vi "MakeTimestampedSegmentExample.vi"() -> ()   [LabVIEW 2015]
uses:
  <vilib>/MDSplus/Library/MDSplus.lvlib
panel:
  out "output array":dbl[][](array[numeric])
  out "MDSplus error":errorcluster
  in  "Samples per segment":i32=100
  in  "Sampling time [ms]":i32=10
  in  "stop":bool
  in  "Phase":dbl
  in  "Amplitude":dbl=5.0
  in  "Frequency":dbl=0.01
  in  "Node path":string
  in  "Run number":i32
  in  "Tree name":string
  # "Before running this example make sure to set the Tree name, Run number and Node path to meaningful values.\nNote that the example does not create a tree structure for you. If a signal (?) node is not already present when you call it, the example will fail."
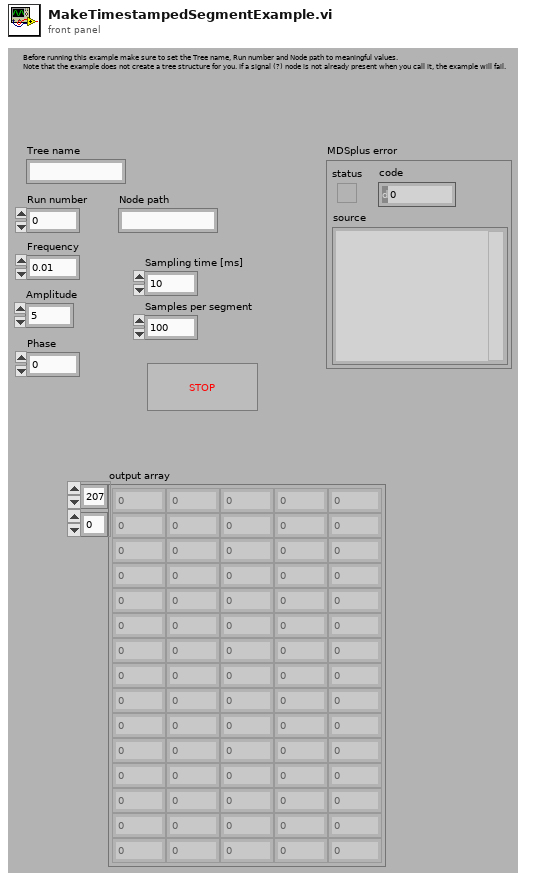
[diagram p1: front panel]
types:
  T1 = cluster{"Data channels":dbl[][], "Timestamps":timestamp[]}
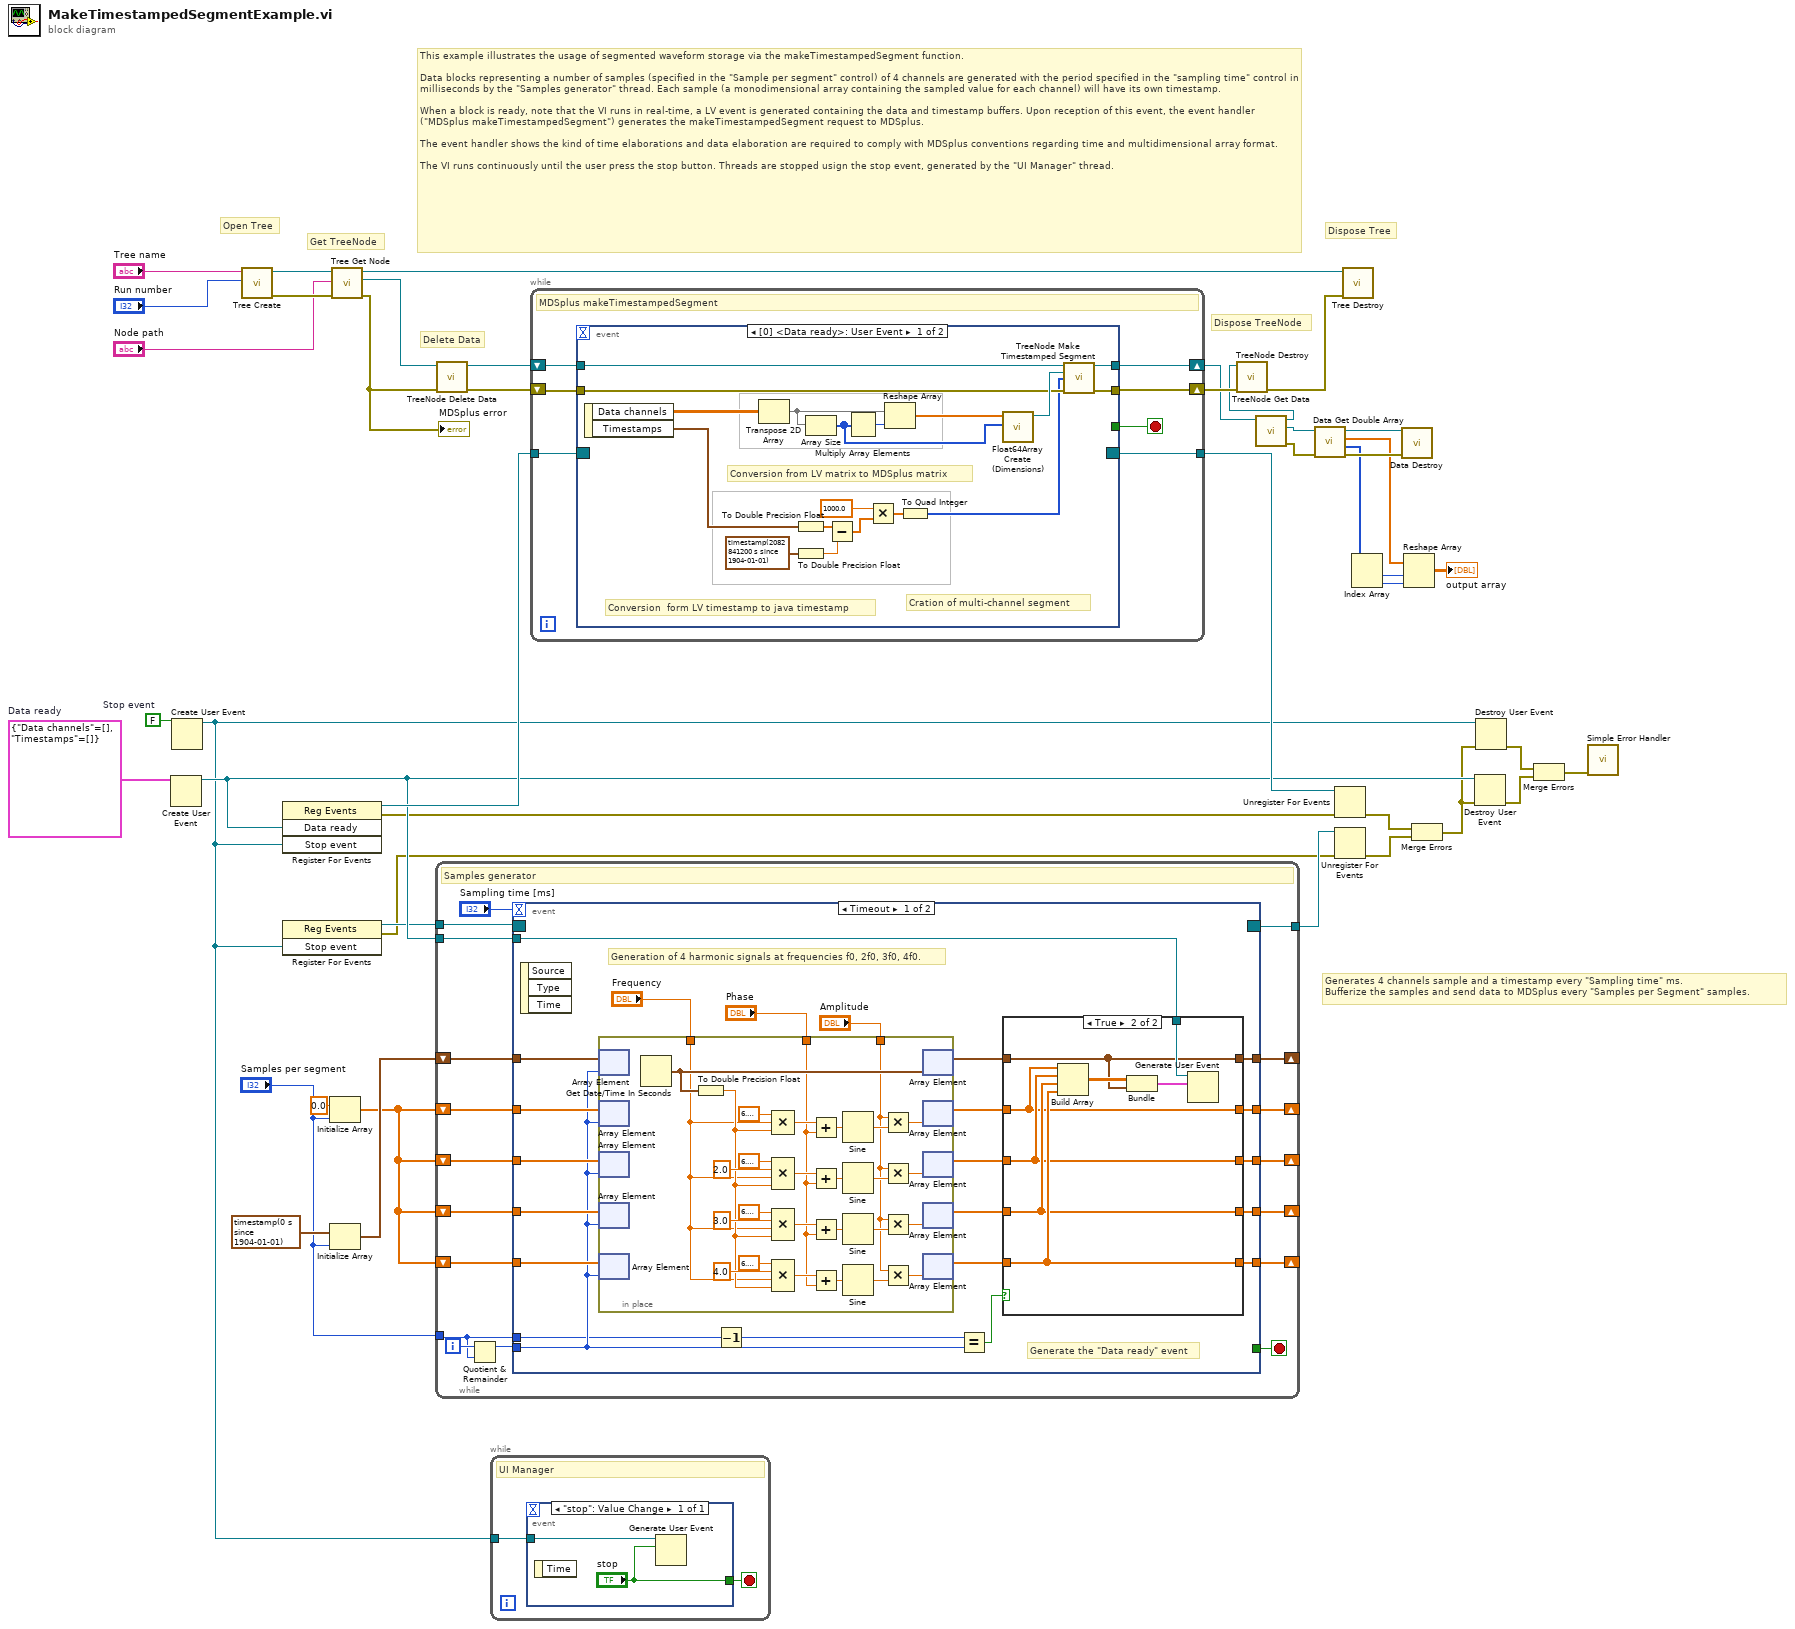
[diagram p0: block diagram]
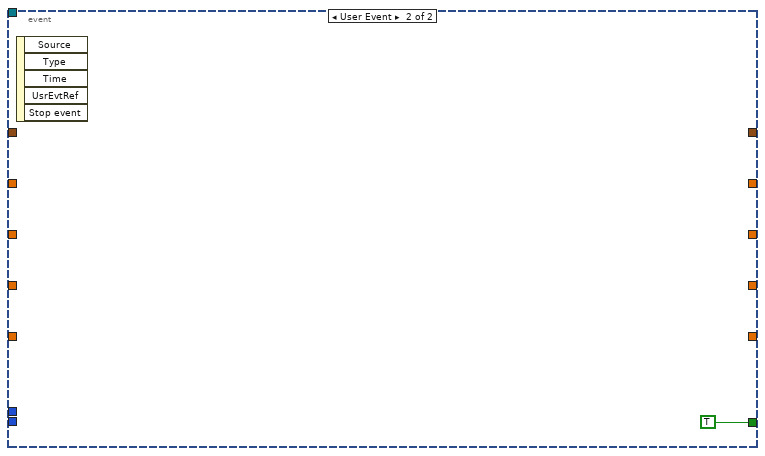
[diagram p3: hidden frame]
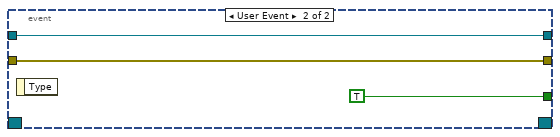
[diagram p4: hidden frame]
diagram:
  w29 = T1 {"Data channels"=[], "Timestamps"=[]}  # Data ready
  w32 = FALSE  # Stop event
  # "Generates 4 channels sample and a timestamp every \"Sampling time\" ms.\nBufferize the samples and send data to MDSplus every \"Samples per Segment\" samples."
  # "Dispose TreeNode"
  # "Delete Data"
  # "Get TreeNode"
  # "This example illustrates the usage of segmented waveform storage via the makeTimestampedSegment function.\n\nData blocks representing a number of samples (specified in the \"Sample per segment\" control) of 4 channels are generated with the period specified in the \"sampling time\" control in milliseconds by the \"Samples generator\" thread. Each sample (a monodimensional array containing the sampled value for each channel) will have its own timestamp.\n\nWhen a block is ready, note that the VI runs in real-time, a LV event is generated containing the data and timestamp buffers. Upon reception of this event, the event handler (\"MDSplus makeTimestampedSegment\") generates the makeTimestampedSegment request to MDSplus.\n\nThe event handler shows the kind of time elaborations and data elaboration are required to comply with MDSplus conventions regarding time and multidimensional array format.\n\nThe VI runs continuously until the user press the stop button. Threads are stopped usign the stop event, generated by the \"UI Manager\" thread."
  # "Dispose Tree"
  # "Open Tree"
  n1 = Create User Event(user event datatype=w29) -> (user event=w33:refnum<user-event>)  [unwired: 1 in, 1 out]
  n2 = Create User Event(user event datatype=w32) -> (user event=w21:refnum<user-event>)  [unwired: 1 in, 1 out]
  n3 = call <vilib>:"Tree Create.vi"("Shot"="Run number", "Name"="Tree name") -> ("error out"=w40:errorcluster, "Tree DVR out"=w42:refnum<data-value>)  [unwired: 8 in]
  n4 = register-events(w33, w21) -> (reference out=w35:refnum<event-registration>, error out=w28:errorcluster)  [unwired: 2 in]
  n5 = register-events(w21) -> (reference out=w25:refnum<event-registration>, error out=w23:errorcluster)  [unwired: 2 in]
  n6 = Initialize Array(0.0 ("phase"), "Samples per segment") -> (w19:dbl[])
  n7 = Initialize Array(timestamp(0 s since 1904-01-01), "Samples per segment") -> (w20:timestamp[])
  n8 = call <vilib>:"Tree Get Node.vi"("error in (no error)"=w40, "Path"="Node path", "Tree DVR in"=w42) -> ("error out"=w13:errorcluster, "Node out"=w37:refnum<data-value>, "Tree DVR out"=w41:refnum<data-value>)  [unwired: 6 in]
  "MDSplus error" <- w13
  n9 = while {
    tunnel: w33 -> [w62]
    shift-right: [w49] -> _
    shift-left: w20 -> [w61]
    shift-right: [w48] -> _
    shift-left: w19 -> [w60]
    shift-right: [w51] -> _
    shift-left: w19 -> [w58]
    shift-right: [w50] -> _
    shift-left: w19 -> [w59]
    shift-right: [w52] -> _
    shift-left: w19 -> [w57]
    tunnel: "Samples per segment" -> [w53]
    tunnel: w25 -> [w47]
    tunnel: [w45] -> w24
    i -> [w56]
    stop <- w46 stop-if-true
    # "Samples generator"
    n10 = Quotient & Remainder(x=w56, y=w53) -> (x-y*floor(x/y)=w55:i32)  [unwired: 1 out]
    n11 = event shown="[0] Timeout" {
      selector: w47 -> [_ _]
      dyn-events: [_ _] -> w45
      timeout: "Sampling time [ms]" -> [_ _]
      tunnel: w62 -> [w80 _]
      tunnel: w61 -> [w79 _]
      tunnel: w60 -> [w78 _]
      tunnel: w59 -> [w77 _]
      tunnel: w58 -> [w76 _]
      tunnel: w57 -> [w75 _]
      tunnel: w55 -> [w71 _]
      tunnel: w53 -> [w64 _]
      tunnel: [w69 _] -> w52
      tunnel: [w68 _] -> w51
      tunnel: [w67 _] -> w50
      tunnel: [w66 _] -> w49
      tunnel: [w65 _] -> w48
      tunnel: [_ TRUE] -> w46
      event Timeout {
        # "Generate the \"Data ready\" event"
        # "Generation of 4 harmonic signals at frequencies f0, 2f0, 3f0, 4f0."
        n12 = event-data() -> ()  [unwired: 1 in, 3 out]
        n13 = in-place {
          in-place-border: "Frequency" -> [w99]
          in-place-border: "Amplitude" -> [w101]
          in-place-border: "Phase" -> [w100]
          n14 = in-place-array #1(w79, w71) -> ()  [unwired: 1 out]
          n15 = in-place-array #2(w78, w71) -> ()  [unwired: 1 out]
          n16 = in-place-array #3(w77, w71) -> ()  [unwired: 1 out]
          n17 = in-place-array #4(w76, w71) -> ()  [unwired: 1 out]
          n18 = in-place-array #5(w75, w71) -> ()  [unwired: 1 out]
          n19 = Get Date/Time In Seconds() -> (seconds since 1Jan1904=w122:timestamp)
          n20 = To Double Precision Float(number=w122) -> (double precision float=w105:dbl)
          n21 = Compound Arithmetic op=MULTIPLY(6.283185307179586, w99, w105) -> (w125:dbl)
          n22 = Compound Arithmetic op=MULTIPLY(6.283185307179586, 2.0 ("value"), w99, w105) -> (w119:dbl)
          n23 = Compound Arithmetic op=MULTIPLY(6.283185307179586, 3.0 ("value"), w99, w105) -> (w114:dbl)
          n24 = Compound Arithmetic op=MULTIPLY(6.283185307179586, 4.0 ("value"), w99, w105) -> (w109:dbl)
          n25 = Add(x=w125, y=w100) -> (x+y=w126:dbl)
          n26 = Add(x=w119, y=w100) -> (x+y=w120:dbl)
          n27 = Add(x=w114, y=w100) -> (x+y=w115:dbl)
          n28 = Add(x=w109, y=w100) -> (x+y=w110:dbl)
          n29 = Sine(x=w126) -> (sin(x)=w124:dbl)
          n30 = Sine(x=w120) -> (sin(x)=w118:dbl)
          n31 = Sine(x=w115) -> (sin(x)=w113:dbl)
          n32 = Sine(x=w110) -> (sin(x)=w108:dbl)
          n33 = Multiply(x=w101, y=w124) -> (x*y=w121:dbl)
          n34 = Multiply(x=w101, y=w118) -> (x*y=w104:dbl)
          n35 = Multiply(x=w101, y=w113) -> (x*y=w103:dbl)
          n36 = Multiply(x=w101, y=w108) -> (x*y=w102:dbl)
          n37 = in-place-array #1(w122) -> (w81:timestamp[])  [unwired: 1 out]
          n38 = in-place-array #2(w121) -> (w82:dbl[])  [unwired: 1 out]
          n39 = in-place-array #3(w104) -> (w83:dbl[])  [unwired: 1 out]
          n40 = in-place-array #4(w103) -> (w84:dbl[])  [unwired: 1 out]
          n41 = in-place-array #5(w102) -> (w85:dbl[])  [unwired: 1 out]
        }
        n42 = Decrement(x=w64) -> (x-1=w63:i32)
        n43 = Equal?(x=w63, y=w71) -> (x = y?=w70:bool)
        n44 = case shown="True" w70 {
          tunnel: w85 -> [w86 w95]
          tunnel: w84 -> [w87 w94]
          tunnel: w83 -> [w88 w93]
          tunnel: w82 -> [w89 w91]
          tunnel: w81 -> [w90 w92]
          tunnel: w80 -> [_ w96]
          tunnel: [w86 w95] -> w69
          tunnel: [w87 w94] -> w68
          tunnel: [w88 w93] -> w67
          tunnel: [w90 w92] -> w66
          tunnel: [w89 w91] -> w65
          frame False {
          }
          frame True {
            n45 = Build Array(w91, w93, w94, w95) -> (w98:dbl[][])
            n46 = Bundle(w98, w92) -> (w97:cluster{dbl[][], timestamp[]})  [unwired: 1 in]
            n47 = Generate User Event(user event=w96, event data cluster=w97) -> ()  [unwired: 2 in, 2 out]
          }
        }
      }
      event User Event {
        n48 = event-data() -> ()  [unwired: 1 in, 5 out]
      }
    }
  }
  n49 = call <vilib>:"TreeNode Delete Data.vi"("error in (no error)"=w13, "TreeNode DVR in"=w37) -> ("error out"=w31:errorcluster, "TreeNode DVR out"=w36:refnum<data-value>)  [unwired: 8 in]
  n50 = while {
    tunnel: w21 -> [w128]
    stop <- w129 stop-if-true
    # "UI Manager"
    n51 = event shown="[0] \"stop\": Value Change" {
      selector: _ -> [_]
      dyn-events: _ -> [_]
      timeout: _ -> [_]
      tunnel: ["stop"] -> w129
      tunnel: w128 -> [w130]
      event "stop": Value Change {
        n52 = event-data() -> ()  [unwired: 1 in, 1 out]
        n53 = Generate User Event(user event=w130, event data cluster="stop") -> ()  [unwired: 2 in, 2 out]
      }
    }
  }
  n54 = while {
    shift-right: [w135] -> w11
    shift-left: w36 -> [w136]
    shift-right: [w132] -> w30
    shift-left: w31 -> [w133]
    tunnel: w35 -> [w138]
    tunnel: [w137] -> w34
    stop <- w134 stop-if-true
    # "MDSplus makeTimestampedSegment"
    n55 = event shown="[0] <Data ready>: User Event" {
      selector: w138 -> [_ _]
      dyn-events: [_ _] -> w137
      timeout: _ -> [_ _]
      tunnel: w136 -> [w156 w157]
      tunnel: [w155 w157] -> w135
      tunnel: w133 -> [w152 w158]
      tunnel: [w154 w158] -> w132
      tunnel: [_ TRUE] -> w134
      event User Event {
        # "Conversion from LV matrix to MDSplus matrix"
        # "Conversion  form LV timestamp to java timestamp"
        # "Cration of multi-channel segment"
        n56 = event-data() -> ("Data channels"=w149:dbl[][], "Timestamps"=w140:timestamp[])  [unwired: 1 in]
        n57 = Transpose 2D Array(2D array=w149) -> (transposed array=w151:dbl[][])
        n58 = To Double Precision Float(number=w140) -> (double precision float=w144:dbl[])
        n59 = To Double Precision Float(number=timestamp(2082841200 s since 1904-01-01)) -> (double precision float=w143:dbl)
        n60 = Array Size(array=w151) -> (size(s)=w147:i32[])
        n61 = Subtract(x=w144, y=w143) -> (x-y=w145:dbl[])
        n62 = Multiply Array Elements(1:w147) -> (0:w150:i32)
        n63 = Multiply(x=1000.0 ("phase"), y=w145) -> (x*y=w146:dbl[])
        n64 = Reshape Array(w151, w150) -> (w148:dbl[])
        n65 = To Quad Integer(1:w146) -> (0:w139:i64[])
        n66 = call <vilib>:"Float64Array Create (Dimensions).vi"("Array dimensions"=w147, "DBL array in"=w148) -> ("Float64Array DVR out"=w153:refnum<data-value>)  [unwired: 8 in, 1 out]
        n67 = call <vilib>:"TreeNode Make Timestamped Segment.vi"("TreeNode DVR in"=w156, "Segment Data DVR"=w153, "Timestamps"=w139, "error in (no error)"=w152) -> ("TreeNode DVR out"=w155:refnum<data-value>, "error out"=w154:errorcluster)  [unwired: 10 in]
      }
      event User Event {
        n68 = event-data() -> ()  [unwired: 1 in, 1 out]
      }
    }
  }
  n69 = call <vilib>:"TreeNode Get Data.vi"("TreeNode DVR in"=w11) -> ("error out"=w8:errorcluster, "Data out"=w12:refnum<data-value>, "TreeNode DVR out"=w10:refnum<data-value>)  [unwired: 8 in]
  n70 = call <vilib>:"TreeNode Destroy.vi"("error in (no error)"=w30, "TreeNode DVR in"=w10) -> ("error out"=w39:errorcluster)  [unwired: 9 in]
  n71 = call <vilib>:"Data Get Double Array.vi"("error in (no error)"=w8, "Data DVR in"=w12) -> ("error out"=w7:errorcluster, "Array dimensions"=w6:i32[], "DBL array out"=w4:dbl[], "Data DVR out"=w9:refnum<data-value>)  [unwired: 6 in]
  n72 = Unregister For Events(event registration refnum=w34, error in=w28) -> (error out=w18:errorcluster)
  n73 = Unregister For Events(event registration refnum=w24, error in=w23) -> (error out=w17:errorcluster)
  n74 = call <vilib>:"Tree Destroy.vi"("error in (no error)"=w39, "Tree DVR in"=w41) -> ()  [unwired: 9 in, 1 out]
  n75 = Index Array(array=w6) -> (element #1=w3:i32, element #2=w2:i32)  [unwired: 2 in]
  n76 = call <vilib>:"Data Destroy.vi"("error in (no error)"=w7, "Data DVR in"=w9) -> ()  [unwired: 9 in, 1 out]
  n77 = Reshape Array(w4, w3, w2) -> (→"output array":dbl[][])
  n78 = Merge Errors(w18, w17) -> (w22:errorcluster)
  n79 = Destroy User Event(user event=w33, error in=w22) -> (error out=w15:errorcluster)
  n80 = Destroy User Event(user event=w21, error in=w22) -> (error out=w16:errorcluster)
  n81 = Merge Errors(w16, w15) -> (w14:errorcluster)
  n82 = call <vilib>:"Simple Error Handler.vi"("error in (no error)"=w14) -> ()  [unwired: 4 in, 5 out]
